vi "ExTestPutI32.vi"() -> ()   [LabVIEW 2010]
panel:
  out "Image Display 2":i32[][](graph)
  out "error out":errorcluster
  in  "error in (no error)":errorcluster
  out "Image Display":i32[][](graph)
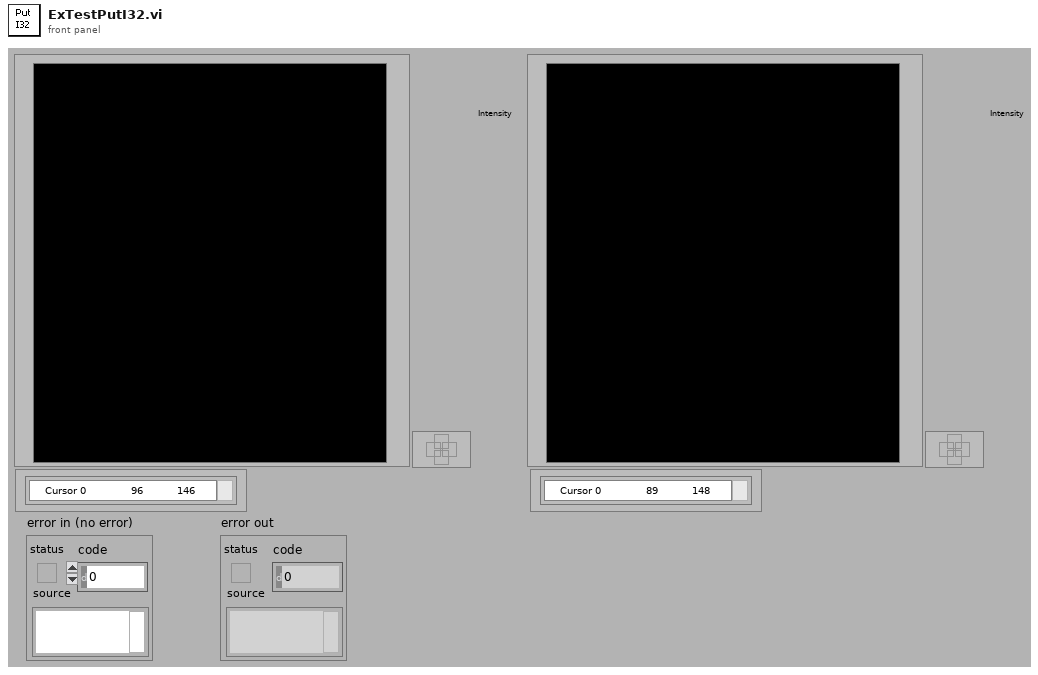
[diagram p1: front panel]
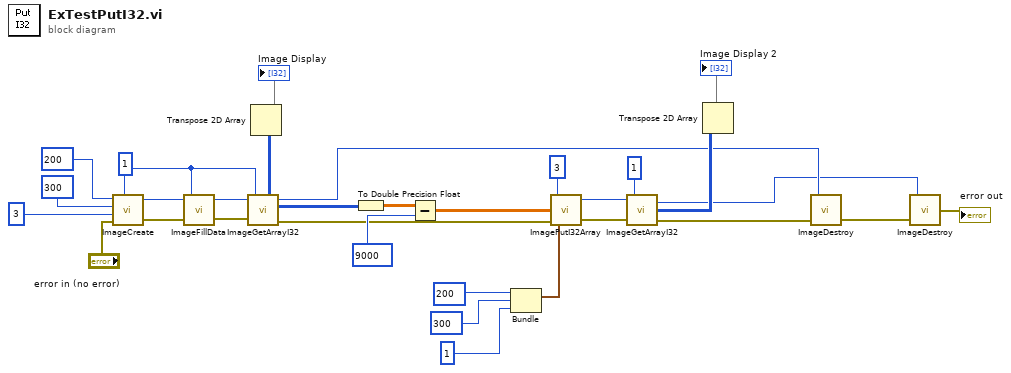
[diagram p0: block diagram]
diagram:
  w21 = 1
  n1 = call <userlib>:"ImageCreate.vi"("X dimension"=200, "Y dimension"=300, "Data Type"=3, "error in"="error in (no error)", "Number Of Frames"=w21) -> ("Image Handle"=w25:u32, "error out"=w26:errorcluster)
  n2 = call <userlib>:"ImageFillData.vi"("error in"=w26, "Type of Test"=w21, "Image Handle"=w25) -> ("error out"=w24:errorcluster, "Image Handle"=w23:u32)
  n3 = call <userlib>:"ImageGetArrayI32.vi"("error in"=w24, "Z position"=w21, "Image Handle"=w23) -> ("error out"=w15:errorcluster, "Array int 32"=w19:i32[][], "Image Handle"=w9:u32)
  n4 = Transpose 2D Array(2D array=w19) -> (transposed array=→"Image Display":i32[][])
  n5 = To Double Precision Float(number=w19) -> (double precision float=w18:dbl[][])
  n6 = Subtract(x=w18, y=9000) -> (x-y=w16:dbl[][])
  n7 = Bundle(200, 300, 1) -> (w4:cluster{i32, i32, i32})  [unwired: 1 in]
  n8 = call <userlib>:"ImagePutI32Array.vi"("error in (no error)"=w15, "Data Type to store as"=3, "Image dimensions"=w4, "Image Data"=w16) -> ("error out"=w14:errorcluster, "Image Handle"=w13:u32)
  n9 = call <userlib>:"ImageGetArrayI32.vi"("error in"=w14, "Z position"=1, "Image Handle"=w13) -> ("error out"=w8:errorcluster, "Array int 32"=w11:i32[][], "Image Handle"=w6:u32)
  n10 = Transpose 2D Array(2D array=w11) -> (transposed array=→"Image Display 2":i32[][])
  n11 = call <userlib>:"ImageDestroy.vi"("error in"=w8, "Data handle"=w9) -> ("error out"=w7:errorcluster)
  n12 = call <userlib>:"ImageDestroy.vi"("error in"=w7, "Data handle"=w6) -> ("error out"=→"error out":errorcluster)
